vi "Set button status.vi"(8 "error in (no error)":errorcluster, 9 "Home?":bool, 10 "End?":bool, 11 "Refnums":T1) -> (0 "error out":errorcluster)   [LabVIEW 2020]
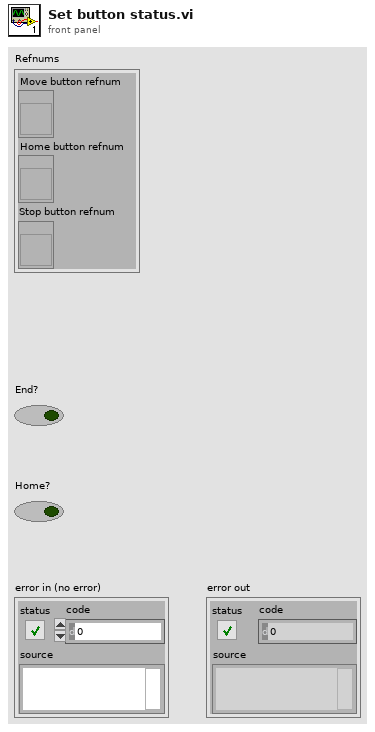
[diagram p1: front panel]
types:
  T1 = typedef "Control references -- typedef.ctl" = cluster{"Move button refnum":refnum<vi>, "Home button refnum":refnum<vi>, "Stop button refnum":refnum<vi>}
  T2 = enum8{"Enabled", "Disabled", "Disabled and Grayed Out"}
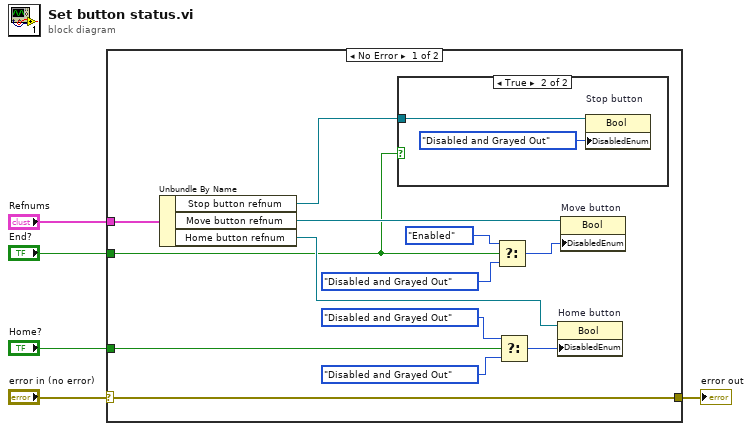
[diagram p0: block diagram]
diagram:
  n1 = case shown="No Error" "error in (no error)" {
    selector: "error in (no error)" -> [w11 w21]
    tunnel: "Refnums" -> [w14 _]
    tunnel: [w11 w21] -> w4
    tunnel: "Home?" -> [w10 _]
    tunnel: "End?" -> [w6 _]
    frame No Error {
      n2 = Unbundle By Name(w14) -> ("Stop button refnum"=w7:refnum<vi>, "Move button refnum"=w13:refnum<vi>, "Home button refnum"=w12:refnum<vi>)
      n3 = case shown="True" w6 {
        tunnel: w7 -> [_ w20]
        frame False {
        }
        frame True {
          n4 = property on="Stop button" class="Bool"(reference=w20, "DisabledEnum"=T2."Disabled and Grayed Out" ("Disabled")) -> ()  [unwired: 1 in, 2 out]
        }
      }
      n5 = Select(t=T2."Enabled" ("Disabled"), s=w6, f=T2."Disabled and Grayed Out") -> (s? t:f=w8:T2)
      n6 = Select(t=T2."Disabled and Grayed Out" ("f"), s=w10, f=T2."Disabled and Grayed Out" ("Disabled")) -> (s? t:f=w9:T2)
      n7 = property on="Home button" class="Bool"(reference=w12, "DisabledEnum"=w9) -> ()  [unwired: 1 in, 2 out]
      n8 = property on="Move button" class="Bool"(reference=w13, "DisabledEnum"=w8) -> ()  [unwired: 1 in, 2 out]
    }
    frame Error {
    }
  }
  "error out" <- w4
